vi "Program Commands.vi"(8 "error in (no error)":errorcluster, 9 "Line/File Number (1)":i32=1 min=1 max=32767, 10 "Command (0:EDIT)":u32(ring) items=["EDIT", "CAT", "LOAD", "STORE", "PURGE", "SCRATCH", "RUN", "STOP", "PAUSE", "CONT", "STEP", "QUIT"], 11 "VISA resource name":refnum<visa-resource-name>) -> (0 "error out":errorcluster, 3 "VISA resource name out":refnum<visa-resource-name>)   [LabVIEW 2010, in "Agilent 4194.lvlib"]
doc: "This function sends BASIC program commands to instrument."
uses:
  <instrlib>/Agilent 4194/Agilent 4194.lvlib
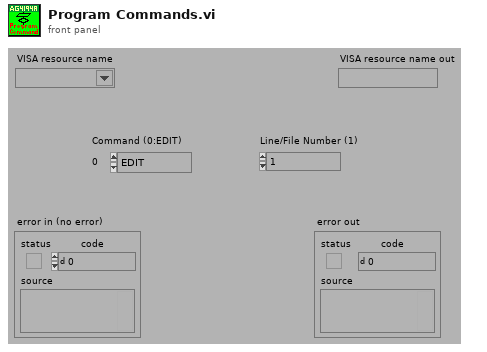
[diagram p1: front panel]
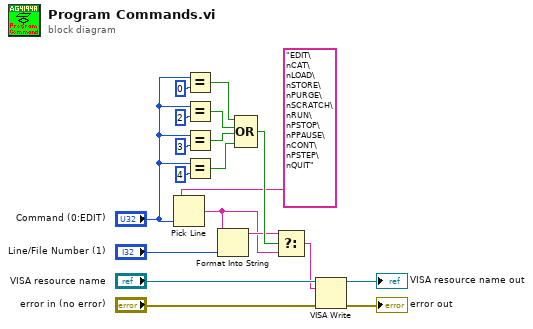
[diagram p0: block diagram]
diagram:
  n1 = Pick Line(multi-line string="EDIT\nCAT\nLOAD\nSTORE\nPURGE\nSCRATCH\nRUN\nPSTOP\nPPAUSE\nCONT\nPSTEP\nQUIT", line index="Command (0:EDIT)") -> (output string=w2:string)  [unwired: 1 in]
  n2 = Equal?(x="Command (0:EDIT)", y=u32 0) -> (x = y?=w10:bool)
  n3 = Equal?(x="Command (0:EDIT)", y=u32 2) -> (x = y?=w9:bool)
  n4 = Equal?(x="Command (0:EDIT)", y=u32 3) -> (x = y?=w8:bool)
  n5 = Equal?(x="Command (0:EDIT)", y=u32 4) -> (x = y?=w7:bool)
  n6 = Format Into String(initial string=w2, "Line/File Number (1)") -> (resulting string=w3:string)  [unwired: 2 in, 1 out]
  n7 = Compound Arithmetic op=OR(w10, w9, w8, w7) -> (w6:bool)
  n8 = Select(t=w3, s=w6, f=w2) -> (s? t:f=w1:string)
  n9 = VISA Write(VISA resource name="VISA resource name", write buffer=w1, error in (no error)="error in (no error)") -> (VISA resource name out=→"VISA resource name out":refnum<visa-resource-name>, error out=→"error out":errorcluster)  [unwired: 1 out]
